vi "Apply best shape.vi"(8 "error in (no error)":errorcluster, 11 "RSA in":refnum<class "RSA.lvclass">) -> (0 "error out":errorcluster, 3 "RSA out":refnum<class "RSA.lvclass">)   [LabVIEW 2012, in "RSA.lvclass"]
uses:
  RSA.lvclass
  RSA.lvclass/RSA.ctl
  <vilib>/Distrio/Murmex/Murmex/Murmex.lvclass
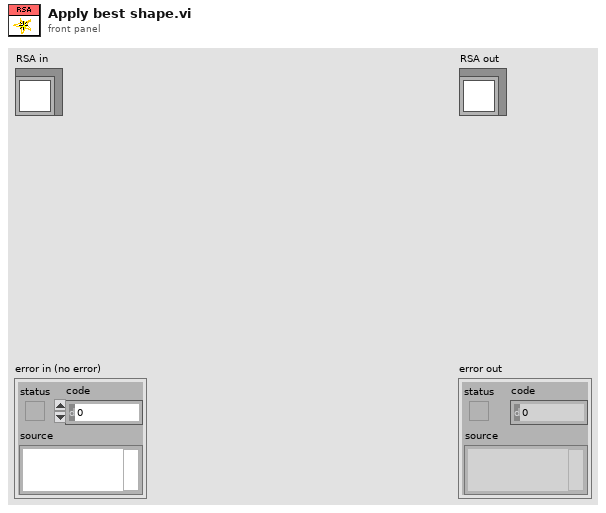
[diagram p1: front panel]
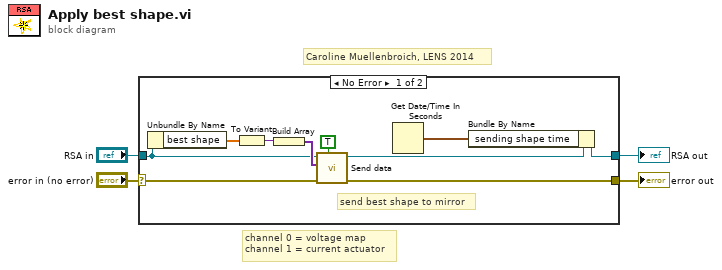
[diagram p0: block diagram]
diagram:
  # "channel 0 = voltage map\nchannel 1 = current actuator"
  # "Caroline Muellenbroich, LENS 2014"
  n1 = case shown="No Error" "error in (no error)" {
    selector: "error in (no error)" -> [w9 w16]
    tunnel: [w8 w16] -> w3
    tunnel: [w6 w15] -> w1
    tunnel: "RSA in" -> [w10 w15]
    frame No Error {
      # "send best shape to mirror"
      n2 = Unbundle By Name(w10) -> ("best shape"=w11:dbl[])
      n3 = To Variant(anything=w11) -> (Variant=w14:variant)
      n4 = Build Array(w14) -> (w13:variant[])
      n5 = call <vilib>:"Send data.vi"("is finalised data? (T)"=TRUE, "error in (no error)"=w9, "data (channels array)"=w13, "Murmex in"=w10) -> ("error out"=w8:errorcluster, "Murmex out"=w7:refnum<class "RSA.lvclass">)  [unwired: 6 in]
      n6 = Get Date/Time In Seconds() -> (seconds since 1Jan1904=w5:timestamp)
      n7 = Bundle By Name(cluster=w7, "sending shape time"=w5) -> (w6:refnum<class "RSA.lvclass">)
    }
    frame Error {
    }
  }
  "error out" <- w3
  "RSA out" <- w1
